vi "Get Type.vi"(8 "error in (no error)":errorcluster, 11 "Project Instr in":refnum<class "Project Instr.lvclass">) -> (0 "error out":errorcluster, 2 "Type":string, 3 "Project Instr out":refnum<class "Project Instr.lvclass">)   [LabVIEW 2015, in "Item Actor.lvlib" / "Project Instr.lvclass"]
uses:
  Project Instr.lvclass
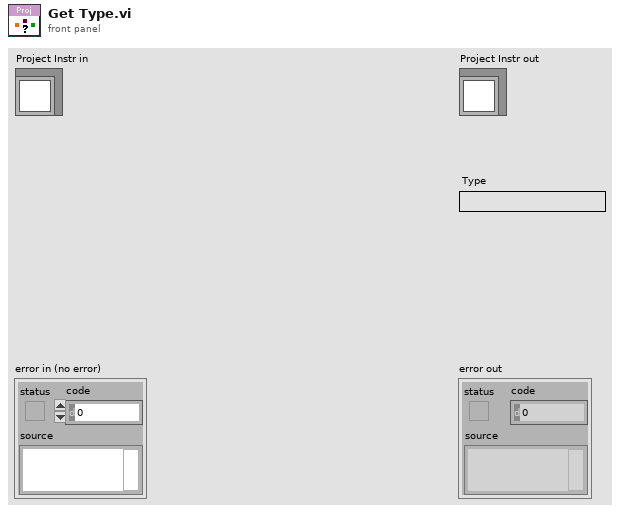
[diagram p1: front panel]
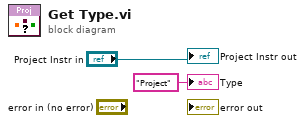
[diagram p0: block diagram]
diagram:
  "Project Instr out" <- "Project Instr in"
  "Type" <- "Project" ("Type")
